vi "stepper44.vi"() -> ()   [LabVIEW 2018]
uses:
  <vilib>/Platform/TimedLoop/XDataNode/timing_clust.ctl
  <vilib>/Platform/TimedLoop/XDataNode/nitl_modes.ctl
  <vilib>/Platform/TimedLoop/XDataNode/wakeup.ctl
  <vilib>/FPGAPlugInAG/myRIO-1900/niLvFpga_Open_myRIO-1900.vi
  <vilib>/rvi/interface/common/dynamic/niFpgaDynamicAddResources.vi
  <vilib>/Utility/error.llb/Error Cluster From Error Code.vi
  <vilib>/rvi/errors/niLvFpgaAdjustHostInterfaceError.vi
  <vilib>/rvi/interface/nirviOpenFPGA/nirviOpenFPGA.xnode
  FPGA Bitfiles/Dentalrobot_FPGATarget_1DIOBoardTestFPG_Hns6xIf0z6s.lvbitx
  FPGA/FPGA_Dental robot.vi
  <vilib>/rvi/interface/nirviReadWriteControl/nirviReadWriteControl.xnode
  <vilib>/Platform/TimedLoop/XDataNode/XDataNode.xnode
  <vilib>/Platform/TimedLoop/XDataNode/XDNodeRunTimeDep.lvlib
  <vilib>/rvi/interface/Simulation/niFpgaSimulationCallBeginRW.vi
  NiFpgaLv.dll
panel:
  out "Cluster":T1
  in  "Step":u32 step=400
  in  "steps / round":i64
  in  "rpm":i64=380 min=10 max=1000 step=10
  in  "Dir":bool
  in  "stop":bool
  # "max speed : ~400rpm"
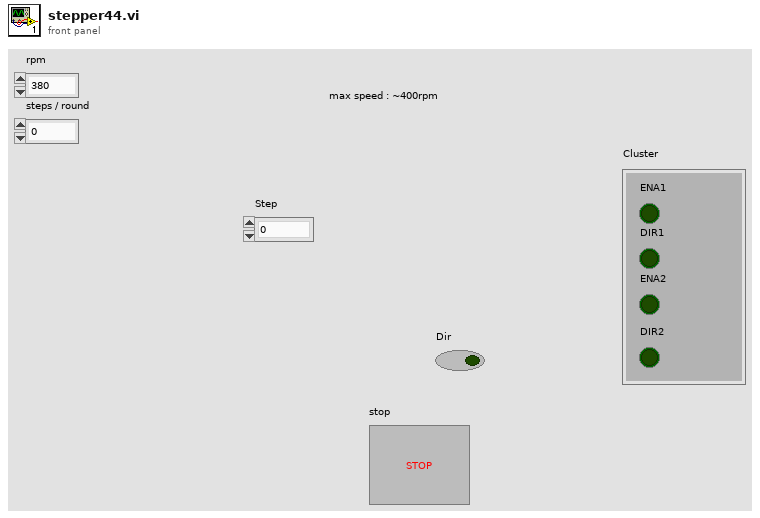
[diagram p1: front panel]
types:
  T1 = cluster{"ENA1":bool, "DIR1":bool, "ENA2":bool, "DIR2":bool}
  T2 = typedef "XDNodeRunTimeDep.lvlib/timing_clust.ctl" = cluster{"Expected End [f-1]":u64, "Actual End [f-1]":u64, "Finished Late? [f-1]":bool, "Expected End [i-1]":u64, "Actual End [i-1]":u64, "Finished Late? [i-1]":bool, "Expected Start [i]":u64, "Actual Start [i]":u64, "Expected Start [f]":u64, "Actual Start [f]":u64, "Source Name":string, "Structure Name":string, "Period":i64, "Deadline":i64, "Offset":i64, "Start":i64, "Priority":i32, "Timeout":i32, "Mode":T3, "Wakeup Reason":T4, "Error":errorcluster, "Source Type":string, "Secondary Source Type":string, "Global End Time":u64, "Global Start Time":u64, "Frame Duration":u64, "Iteration Duration":u64, "Assigned CPU":i32, "I/O Scan Engine Mode":u32}
  T3 = typedef "XDNodeRunTimeDep.lvlib/nitl_modes.ctl" = enum32{"No Change", "Process missed periods, maintain original phase", "Discard missed periods, maintain original phase", "Process missed periods, ignore original phase", "Discard missed periods, ignore original phase"}
  T4 = typedef "XDNodeRunTimeDep.lvlib/wakeup.ctl" = enum32{"Normal", "Aborted", "Asynchronous wakeup", "Timing source error", "Timed loop error", "Timeout"}
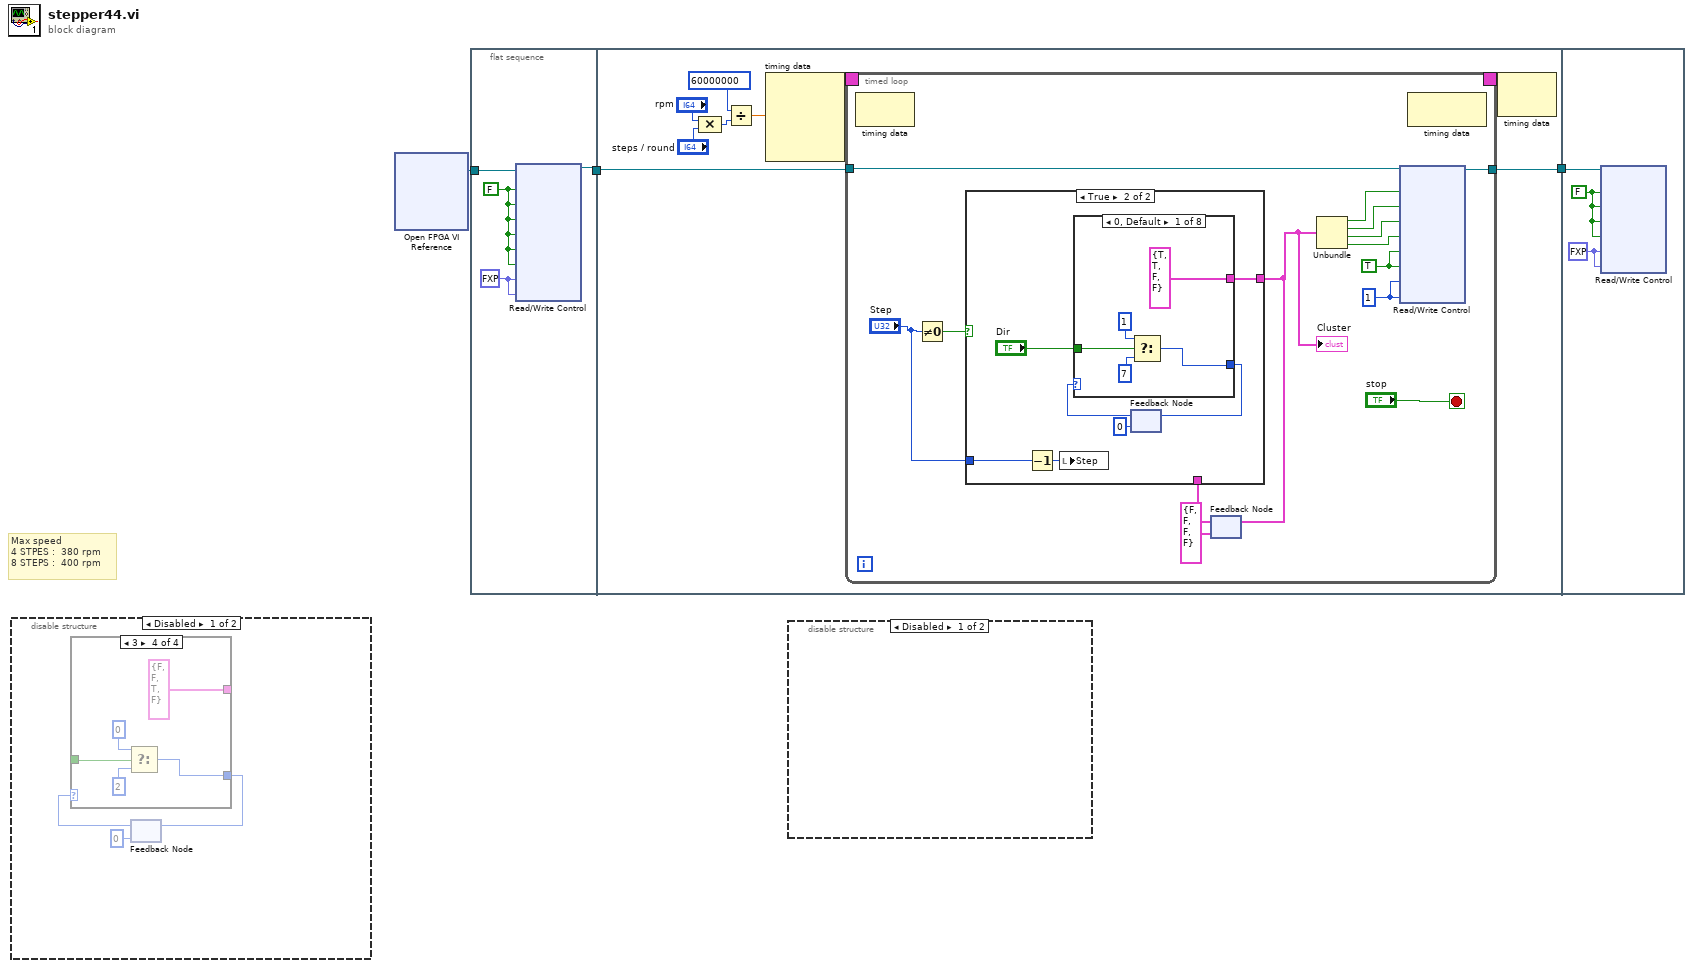
[diagram p0: block diagram]
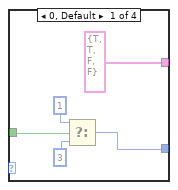
[diagram p3: hidden frame]
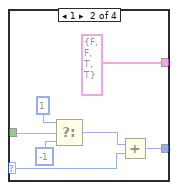
[diagram p4: hidden frame]
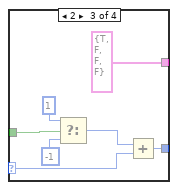
[diagram p5: hidden frame]
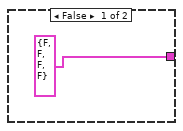
[diagram p7: hidden frame]
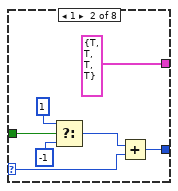
[diagram p8: hidden frame]
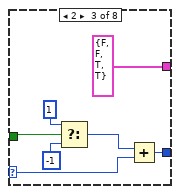
[diagram p9: hidden frame]
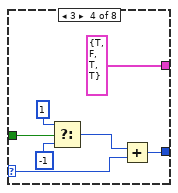
[diagram p10: hidden frame]
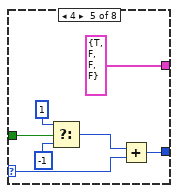
[diagram p11: hidden frame]
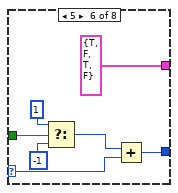
[diagram p12: hidden frame]
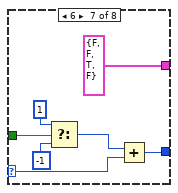
[diagram p13: hidden frame]
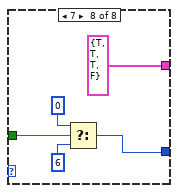
[diagram p14: hidden frame]
diagram:
  # "Max speed\n4 STPES :  380 rpm\n8 STEPS :  400 rpm"
  n1 = disable-structure shown="Disabled" {
    frame Disabled {
      n2 = feedback #1(0) -> (w6:u32)
      n3 = case shown="3" w6 {
        selector: w6 -> [_ w17 w24 _]
        tunnel: [w8 w18 w25 w27] -> w4
        tunnel: _ -> [w11 w14 w21 w28]
        tunnel: [cluster{bool, bool, bool, bool} {TRUE, TRUE, FALSE, FALSE} cluster{bool, bool, bool, bool} {FALSE, FALSE, TRUE, TRUE} cluster{bool, bool, bool, bool} {TRUE, FALSE, FALSE, FALSE} cluster{bool, bool, bool, bool} {FALSE, FALSE, TRUE, FALSE}] -> _
        frame 0, Default {
          n4 = Select(t=1, s=w11, f=3) -> (s? t:f=w8:i32)
        }
        frame 1 {
          n5 = Select(t=1, s=w14, f=-1) -> (s? t:f=w13:i32)
          n6 = Add(x=w13, y=w17) -> (x+y=w18:u32)
        }
        frame 2 {
          n7 = Select(t=1, s=w21, f=-1) -> (s? t:f=w20:i32)
          n8 = Add(x=w20, y=w24) -> (x+y=w25:u32)
        }
        frame 3 {
          n9 = Select(t=0, s=w28, f=2) -> (s? t:f=w27:i32)
        }
      }
      n10 = feedback-in #1(w4) -> ()
    }
    frame Enabled {
    }
  }
  n11 = xnode "Open FPGA VI Reference"() -> ("FPGA VI Reference Out"=w1:refnum<k20>)  [unwired: 2 in, 1 out]
  n12 = flat-sequence {
    tunnel: [w33] -> w2
    tunnel: w1 -> [w31]
    tunnel: [w43] -> w3
    tunnel: w2 -> [w42]
    tunnel: w3 -> [w126]
    frame #0 {
      w32 = fxp<+,32,0> 0.0 ("CH1 DC")
      w34 = FALSE ("ENA1")
      n13 = xnode "Read/Write Control"("FPGA VI Reference In"=w31, "ENA1"=w34, "STBY1"=w34, "DIR1"=w34, "ENA2"=w34, "STBY2"=w34, "DIR2"=w34, "CH1 DC"=w32, "CH2 DC"=w32) -> ("FPGA VI Reference Out"=w33:refnum<k20>)  [unwired: 1 in, 1 out]
    }
    frame #1 {
      n14 = Compound Arithmetic op=MULTIPLY("rpm", "steps / round") -> (w37:i64)
      n15 = Divide(x=i64 60000000, y=w37) -> (x/y=w35:dbl)
      n16 = node-c288(w35) -> (w41:T2)  [unwired: 3 in]
      n17 = timed-loop {
        timing: w41 -> [_]
        timing-out: [_] -> w40
        tunnel: [w56] -> w43
        tunnel: w42 -> [w55]
        stop <- "stop" stop-if-true
        w49 = 1 ("CH1 DC")
        w53 = TRUE ("STBY1")
        n18 = node-c288() -> ()  [unwired: 1 in, 1 out]
        n19 = Not Equal To 0?(x="Step") -> (x != 0?=w48:bool)
        n20 = feedback #2(cluster{bool, bool, bool, bool} {FALSE, FALSE, FALSE, FALSE}) -> (w46:cluster{bool, bool, bool, bool})
        n21 = case shown="True" w48 {
          tunnel: [cluster{bool, bool, bool, bool} {FALSE, FALSE, FALSE, FALSE} w65] -> w44
          tunnel: "Step" -> [_ w59]
          tunnel: w46 -> [_ _]
          frame False {
          }
          frame True {
            n22 = Decrement(x=w59) -> (x-1=w60:u32)
            n23 = local write "Step"(w60) -> ()
            n24 = feedback #3(0) -> (w62:u32)
            n25 = case shown="0, Default" w62 {
              selector: w62 -> [_ w76 w83 w86 w92 w99 w106 _]
              tunnel: [w67 w77 w84 w85 w93 w101 w109 w113] -> w63
              tunnel: "Dir" -> [w70 w73 w80 w87 w94 w100 w107 w114]
              tunnel: [cluster{bool, bool, bool, bool} {TRUE, TRUE, FALSE, FALSE} cluster{bool, bool, bool, bool} {TRUE, TRUE, TRUE, TRUE} cluster{bool, bool, bool, bool} {FALSE, FALSE, TRUE, TRUE} cluster{bool, bool, bool, bool} {TRUE, FALSE, TRUE, TRUE} cluster{bool, bool, bool, bool} {TRUE, FALSE, FALSE, FALSE} cluster{bool, bool, bool, bool} {TRUE, FALSE, TRUE, FALSE} cluster{bool, bool, bool, bool} {FALSE, FALSE, TRUE, FALSE} cluster{bool, bool, bool, bool} {TRUE, TRUE, TRUE, FALSE}] -> w65
              frame 0, Default {
                n26 = Select(t=1, s=w70, f=7) -> (s? t:f=w67:i32)
              }
              frame 1 {
                n27 = Select(t=1, s=w73, f=-1) -> (s? t:f=w72:i32)
                n28 = Add(x=w72, y=w76) -> (x+y=w77:u32)
              }
              frame 2 {
                n29 = Select(t=1, s=w80, f=-1) -> (s? t:f=w79:i32)
                n30 = Add(x=w79, y=w83) -> (x+y=w84:u32)
              }
              frame 3 {
                n31 = Select(t=1, s=w87, f=-1) -> (s? t:f=w88:i32)
                n32 = Add(x=w88, y=w86) -> (x+y=w85:u32)
              }
              frame 4 {
                n33 = Select(t=1, s=w94, f=-1) -> (s? t:f=w96:i32)
                n34 = Add(x=w96, y=w92) -> (x+y=w93:u32)
              }
              frame 5 {
                n35 = Select(t=1, s=w100, f=-1) -> (s? t:f=w103:i32)
                n36 = Add(x=w103, y=w99) -> (x+y=w101:u32)
              }
              frame 6 {
                n37 = Select(t=1, s=w107, f=-1) -> (s? t:f=w110:i32)
                n38 = Add(x=w110, y=w106) -> (x+y=w109:u32)
              }
              frame 7 {
                n39 = Select(t=0, s=w114, f=6) -> (s? t:f=w113:i32)
              }
            }
            n40 = feedback-in #3(w63) -> ()
          }
        }
        "Cluster" <- w44
        n41 = feedback-in #2(w44) -> ()
        n42 = Unbundle(w44) -> (w54:bool, w52:bool, w51:bool, w50:bool)
        n43 = xnode "Read/Write Control"("FPGA VI Reference In"=w55, "ENA1"=w54, "DIR1"=w52, "ENA2"=w51, "DIR2"=w50, "STBY1"=w53, "STBY2"=w53, "CH1 DC"=w49, "CH2 DC"=w49) -> ("FPGA VI Reference Out"=w56:refnum<k20>)  [unwired: 1 in, 1 out]
        n44 = node-c288() -> ()  [unwired: 1 in, 1 out]
      }
      n45 = node-c288(w40) -> ()  [unwired: 1 out]
    }
    frame #2 {
      w124 = fxp<+,32,0> 0.0 ("CH1 DC")
      w125 = FALSE ("ENA1")
      n46 = xnode "Read/Write Control"("FPGA VI Reference In"=w126, "ENA1"=w125, "STBY1"=w125, "ENA2"=w125, "STBY2"=w125, "CH1 DC"=w124, "CH2 DC"=w124) -> ()  [unwired: 1 in, 2 out]
    }
  }
  n47 = disable-structure shown="Disabled" {
    frame Disabled {
    }
    frame Enabled {
    }
  }
